vi "UnevenIntegration.vi"(1 "t":dbl[](array[numeric]), 2 "X":dbl[](array[numeric])) -> (0 "Y":dbl[](array[numeric]))   [LabVIEW 2012]
uses:
  <vilib>/Analysis/NI_AALPro.lvlib
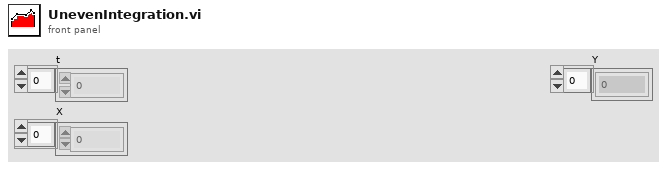
[diagram p1: front panel]
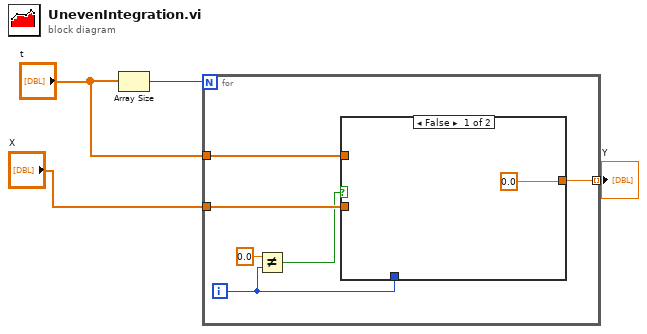
[diagram p0: block diagram]
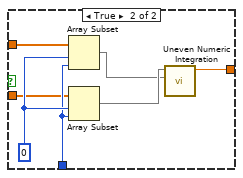
[diagram p2: hidden frame]
diagram:
  n1 = Array Size(array="t") -> (size(s)=w4:i32)
  n2 = for {
    N: w4 -> [_]
    tunnel: "t" -> [w10]
    tunnel: "X" -> [w9]
    tunnel: [w8] -> w1 mode=indexing
    i -> [w5]
    n3 = Not Equal?(x=0.0, y=w5) -> (x != y?=w6:bool)
    n4 = case shown="False" w6 {
      tunnel: w5 -> [_ w17]
      tunnel: w10 -> [_ w16]
      tunnel: w9 -> [_ w15]
      tunnel: [0.0 w12] -> w8
      frame False {
      }
      frame True {
        w18 = 0 ("index")
        n5 = Array Subset(array=w16, index=w18, length=w17) -> (w13:dbl[])
        n6 = Array Subset(array=w15, index=w18, length=w17) -> (w14:dbl[])
        n7 = call <vilib>:"Uneven Numeric Integration.vi"("T"=w13, "X"=w14) -> ("result"=w12:dbl)  [unwired: 8 in, 1 out]
      }
    }
  }
  "Y" <- w1
